vi "EOL CAN_Get Multi Rx.vi"(7 "Rx Arbitration Id":u32=402522244 format="%.0x", 8 "TxRx Data in":string[][](array[string]), 9 "Rx Bytes Length":u8, 11 "data":T1[](array[typedef]) {"payload" format="%x"; "timestamp" format="%<%.7X\n%x>T"; "type" items=["CAN Data"=0, "CAN Remote"=1, "CAN Bus Error"=2, "CAN 2.0 Data"=8, "CAN FD Data"=16, "CAN FD+BRS Data"=24, "J1939 Data"=192, "Delay"=224, "Log Trigger"=225, "Start Trigger"=226]; "identifier" format="%x"}) -> (0 "TxRx Data out":string[][](array[string]), 1 "Response Good?":bool, 2 "Rx Data":u8[](array[numeric]) format="%.0x")   [LabVIEW 2018]
uses:
  <vilib>/xnet/xnet.llb/XNET Frame CAN.ctl
  <vilib>/xnet/xnet.llb/XNET Frame Type CAN.ctl
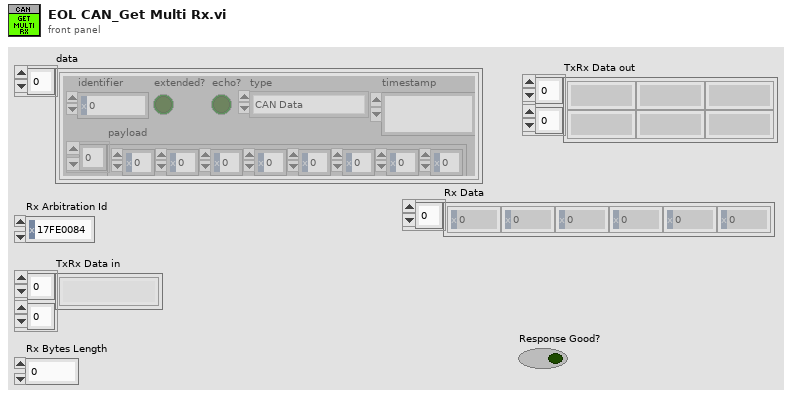
[diagram p1: front panel]
types:
  T1 = typedef "XNET Frame CAN.ctl" = cluster{"timestamp":timestamp, "payload":u8[], "identifier":u32, "type":T2, "extended?":bool, "echo?":bool}
  T2 = typedef "XNET Frame Type CAN.ctl" = u8
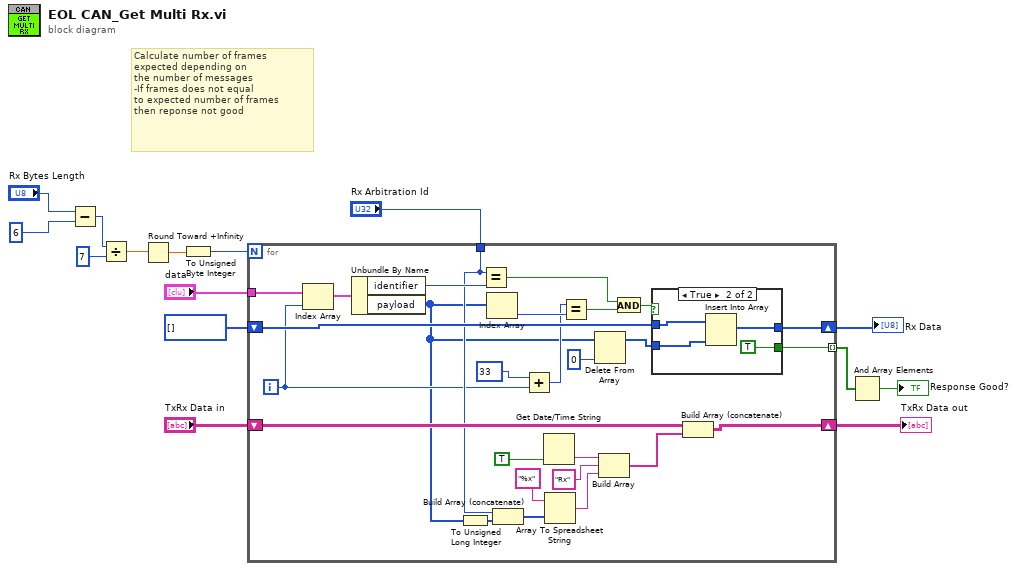
[diagram p0: block diagram]
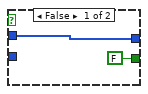
[diagram p2: hidden frame]
diagram:
  # "Calculate number of frames \nexpected depending on\nthe number of messages\n-If frames does not equal\nto expected number of frames\nthen reponse not good"
  n1 = Subtract(x="Rx Bytes Length", y=u8 6) -> (x-y=w6:u8)
  n2 = Divide(x=w6, y=u8 7) -> (x/y=w3:dbl)
  n3 = Round Toward +Infinity(x=w3) -> (ceil(x): smallest int >= x=w2:dbl)
  n4 = To Unsigned Byte Integer(number=w2) -> (unsigned 8bit integer=w4:u8)
  n5 = for {
    N: w4 -> [_]
    shift-right: [w41] -> w1
    shift-left: u8[] [] ("Data Array") -> [w40]
    shift-right: [w27] -> w13
    shift-left: "TxRx Data in" -> [w26]
    tunnel: "data" -> [w22]
    tunnel: "Rx Arbitration Id" -> [w25]
    tunnel: [w23] -> w10 mode=indexing
    i -> [w21]
    n6 = Index Array(array=w22, index=w21) -> (element=w20:T1)
    n7 = Unbundle By Name(w20) -> ("identifier"=w42:u32, "payload"=w18:u8[])
    n8 = To Unsigned Long Integer(number=w18) -> (unsigned 32bit integer=w28:u32[])
    n9 = Equal?(x=w25, y=w42) -> (x = y?=w36:bool)
    n10 = Index Array(array=w18) -> (element=w37:u8)  [unwired: 1 in]
    n11 = Build Array (concatenate)(w25, w28) -> (w29:u32[])
    n12 = Add(x=u8 33, y=w21) -> (x+y=w19:i32)
    n13 = Get Date/Time String(want seconds? (F)=TRUE) -> (time string=w32:string)  [unwired: 2 in, 1 out]
    n14 = Array To Spreadsheet String(array=w29, 3:"%x" ("format string")) -> (spreadsheet string=w34:string)  [unwired: 1 in]
    n15 = Equal?(x=w19, y=w37) -> (x = y?=w38:bool)
    n16 = Delete From Array(array=w18, index=0 ("length")) -> (array with subset deleted=w17:u8[])  [unwired: 1 in, 1 out]
    n17 = Build Array(w32, "Rx" ("format string"), w34) -> (w35:string[])
    n18 = And(x=w36, y=w38) -> (x .and. y?=w39:bool)
    n19 = case shown="True" w39 {
      tunnel: w17 -> [_ w46]
      tunnel: [w44 w45] -> w41
      tunnel: w40 -> [w44 w47]
      tunnel: [FALSE TRUE] -> w23
      frame False {
      }
      frame True {
        n20 = Insert Into Array(array=w47, new element=w46) -> (w45:u8[])  [unwired: 1 in]
      }
    }
    n21 = Build Array (concatenate)(w26, w35) -> (w27:string[][])
  }
  "TxRx Data out" <- w13
  "Rx Data" <- w1
  n22 = And Array Elements(Boolean array=w10) -> (logical AND=→"Response Good?":bool)
